vi "Associate Instruments to Paths.vi"(0 "Scalar SG Path Group in":refnum<class "SG 18GHz Path Group.lvclass">, 5 "TSM Context":T1, 11 "error in (no error)":errorcluster) -> (4 "Scalar SG Path Group out":refnum<class "SG 18GHz Path Group.lvclass">, 15 "error out":errorcluster)   [LabVIEW 2023, in "RFFixtureCharact.RFPM.lvlib" / "SG 18GHz Path Group.lvclass"]
uses:
  SG 18GHz Path Group.lvclass
  C:/srd-semi-rfcal-software/AuxTools/STSRFFixtureCharactUtility/Source/Code Modules/Common/Base Classes/Path Group/Path Group.lvclass
  <vilib>/NI_TestStand_SemiconductorModule/NI_TestStand_Semiconductor_Module.lvlibp/PinMap/General/SemiconductorModuleContext.ctl
  Paths/SG Path/SG 18GHz Path.lvclass
  C:/srd-semi-rfcal-software/AuxTools/STSRFFixtureCharactUtility/Source/Code Modules/Fixture/Public/Base Classes/Scalar/SG Abstract Path/SG Abstract Path.lvclass
  C:/srd-semi-rfcal-software/AuxTools/STSRFFixtureCharactUtility/Source/Code Modules/Common/Base Classes/Path/Path.lvclass
  C:/srd-semi-rfcal-software/AuxTools/STSRFFixtureCharactUtility/Source/Code Modules/Fixture/Public/Base Classes/Scalar/Scalar Path/Scalar Path.lvclass
  Public/Base Classes/Scalar/SG Abstract Path/SG Abstract Path.lvclass
  Charact Result Accessor/Scalar/Scalar Charact Result Accessor.lvclass
  C:/srd-semi-rfcal-software/AuxTools/STSRFFixtureCharactUtility/Source/Code Modules/Fixture/RFPM/Charact Result Accessor/Base/Charact Result Accessor.lvclass
  C:/srd-semi-rfcal-software/AuxTools/STSRFFixtureCharactUtility/Source/Code Modules/Common/Result Accessor/Result Accessor.lvclass
  <vilib>/NI_TestStand_SemiconductorModule/NI_TestStand_Semiconductor_Module.lvlibp/PinMap/RF/RFPM/PinToNIRFPMSessionsWithPaths.vi
  <vilib>/NI_TestStand_SemiconductorModule/NI_TestStand_Semiconductor_Module.lvlibp/PinMap/RF/RFSG/PinToNIRFSGSession.vi
  Common/Base Classes/Path/Path.lvclass
  Common/Result Accessor/Result Accessor.lvclass
  <vilib>/NI_TestStand_SemiconductorModule/NI_TestStand_Semiconductor_Module.lvlibp
  Common/Base Classes/Path Group/Path Group.lvclass
  Instruments/Power Meter/Power Meter Factory/Power Meter Factory.lvclass
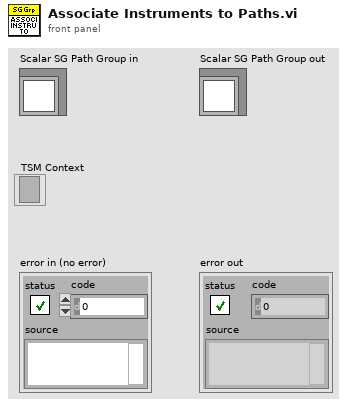
[diagram p1: front panel]
types:
  T1 = typedef "NI_TestStand_Semiconductor_Module.lvlibp/SemiconductorModuleContext.ctl" = refnum<k7>
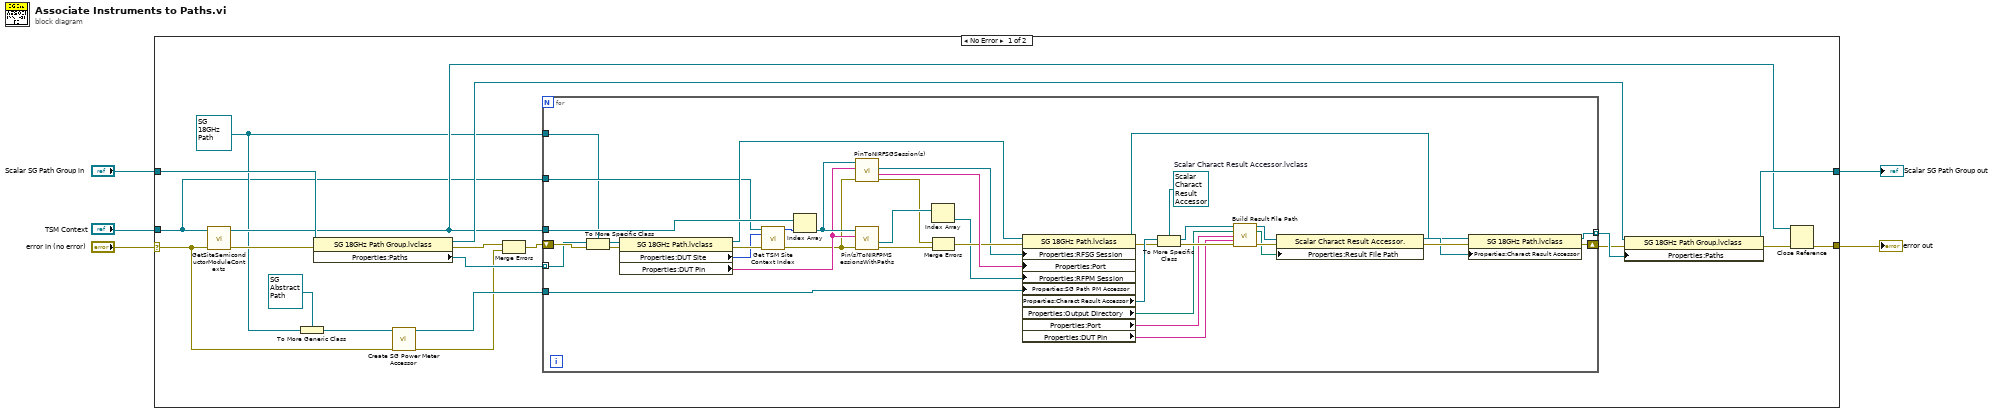
[diagram p0: block diagram]
diagram:
  n1 = case shown="No Error" "error in (no error)" {
    selector: "error in (no error)" -> [w7 w64]
    tunnel: "TSM Context" -> [w8 _]
    tunnel: "Scalar SG Path Group in" -> [w19 w63]
    tunnel: [w18 w64] -> w2
    tunnel: [w20 w63] -> w1
    frame No Error {
      w14 = refnum<class "SG 18GHz Path.lvclass"> refnum ("STS Scalar Fixture Characterization.lvlib:Scalar SG Path.lvclass")
      n2 = call <vilib>:"GetSiteSemiconductorModuleContexts.vi"("error in (no error)"=w7, "Semiconductor Module Context"=w8) -> ("error out"=w23:errorcluster, "Site Semiconductor Module Contexts"=w17:T1[])  [unwired: 8 in]
      n3 = To More Generic Class(target class=refnum<class "SG Abstract Path.lvclass"> refnum ("RFFixtureCharact.Common.lvlib:SG Path.lvclass"), reference=w14) -> (generic class reference=w6:refnum<class "SG Abstract Path.lvclass">)
      n4 = property class="SG 18GHz Path Group.lvclass"(reference=w19, error in=w23) -> (reference out=w22:refnum<class "SG 18GHz Path Group.lvclass">, error out=w12:errorcluster, "Properties:Paths"=w24:refnum<class "Path.lvclass">[])
      n5 = call "Create SG Power Meter Accessor.vi"("SG Path"=w6, "error in"=w7) -> ("SG Path PM Accessor out"=w16:refnum<class "SG Path PM Accessor Base.lvclass">, "error out"=w11:errorcluster)  [unwired: 12 in]
      n6 = Merge Errors(w12, w11) -> (w10:errorcluster)
      n7 = for {
        tunnel: w17 -> [w62]
        tunnel: w24 -> [w49] mode=indexing
        tunnel: [w36] -> w21 mode=indexing
        tunnel: w16 -> [w47]
        tunnel: w8 -> [w42]
        tunnel: w14 -> [w41]
        shift-right: [w35] -> w13
        shift-left: w10 -> [w51]
        w40 = refnum<class "Scalar Charact Result Accessor.lvclass"> refnum  # Scalar Charact Result Accessor.lvclass
        n8 = To More Specific Class(target class=w41, reference=w49, error in=w51) -> (specific class reference=w48:refnum<class "SG 18GHz Path.lvclass">, error out=w50:errorcluster)
        n9 = property class="SG 18GHz Path.lvclass"(reference=w48, error in=w50) -> (reference out=w52:refnum<class "SG 18GHz Path.lvclass">, error out=w54:errorcluster, "Properties:DUT Site"=w44:i32, "Properties:DUT Pin"=w46:string)
        n10 = call "Get TSM Site Context Index.vi"("Semiconductor Module Context"=w42, "Site Number"=w44, "error in (no error)"=w54) -> ("index of Site TSM Context"=w43:i32, "error out"=w45:errorcluster)  [unwired: 11 in]
        n11 = Index Array(array=w62, index=w43) -> (element=w55:T1)
        n12 = call-poly <vilib>:"Pin(s)ToNIRFPMSessionsWithPaths.vi"("error in (no error)"=w45, "Pin"=w46, "Semiconductor Module Context"=w55) -> ("error out"=w58:errorcluster, "Instrument Sessions"=w61:refnum<k15>[])  [unwired: 3 in, 4 out]
        n13 = call-poly <vilib>:"PinToNIRFSGSession(s).vi"("error in (no error)"=w45, "Pin"=w46, "Semiconductor Module Context"=w55) -> ("error out"=w53:errorcluster, "Port"=w60:string, "Instrument Session"=w56:refnum<k15>)  [unwired: 4 in, 2 out]
        n14 = Index Array(array=w61) -> (element=w57:refnum<k15>)  [unwired: 1 in]
        n15 = Merge Errors(w53, w58) -> (w59:errorcluster)
        n16 = property class="SG 18GHz Path.lvclass"(reference=w52, error in=w59, "Properties:RFSG Session"=w56, "Properties:Port"=w60, "Properties:RFPM Session"=w57, "Properties:SG Path PM Accessor"=w47) -> (reference out=w33:refnum<class "SG 18GHz Path.lvclass">, error out=w34:errorcluster, "Properties:Charact Result Accessor"=w37:refnum<class "Result Accessor.lvclass">, "Properties:Output Directory"=w27:path, "Properties:Port"=w26:string, "Properties:DUT Pin"=w25:string)
        n17 = To More Specific Class(target class=w40, reference=w37, error in=w34) -> (specific class reference=w32:refnum<class "Scalar Charact Result Accessor.lvclass">, error out=w31:errorcluster)
        n18 = call-dynamic "Build Result File Path.vi"("Charact Result Accessor in"=w32, "Output Directory"=w27, "Port 1"=w26, "Port 2"=w25, "error in"=w31) -> ("Charact Result Accessor out"=w29:refnum<class "Scalar Charact Result Accessor.lvclass">, "Result File Path"=w28:path, "error out"=w30:errorcluster)  [unwired: 8 in]
        n19 = property class="Scalar Charact Result Accessor."(reference=w29, error in=w30, "Properties:Result File Path"=w28) -> (reference out=w38:refnum<class "Scalar Charact Result Accessor.lvclass">, error out=w39:errorcluster)
        n20 = property class="SG 18GHz Path.lvclass"(reference=w33, error in=w39, "Properties:Charact Result Accessor"=w38) -> (reference out=w36:refnum<class "SG 18GHz Path.lvclass">, error out=w35:errorcluster)
      }
      n21 = property class="SG 18GHz Path Group.lvclass"(reference=w22, error in=w13, "Properties:Paths"=w21) -> (reference out=w20:refnum<class "SG 18GHz Path Group.lvclass">, error out=w9:errorcluster)
      n22 = Close Reference(reference=w17, error in (no error)=w9) -> (error out=w18:errorcluster)
    }
    frame Error {
    }
  }
  "error out" <- w2
  "Scalar SG Path Group out" <- w1
